vi "test json to variant bool.vi"(8 "error in (no error)":errorcluster) -> (0 "error out":errorcluster)   [LabVIEW 2019, in "labview_json_tests.lvlib"]
uses:
  labview_json_tests.lvlib
  lib/labview_json.lvlib
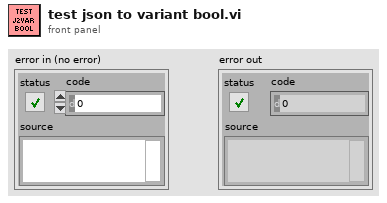
[diagram p1: front panel]
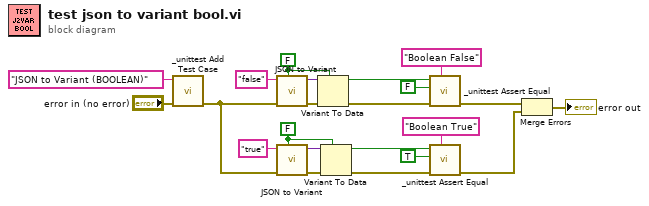
[diagram p0: block diagram]
diagram:
  w2 = FALSE
  w5 = FALSE
  n1 = call "_unittest Add Test Case.vi"("error in (no error)"="error in (no error)", "Test Case"="JSON to Variant (BOOLEAN)") -> ("error out"=w10:errorcluster)  [unwired: 9 in]
  n2 = call "JSON to Variant.vi"("Variant Type"=w5, "error in (no error)"=w10, "JSON"="false") -> ("error out"=w8:errorcluster, "Variant out"=w16:variant)  [unwired: 7 in]
  n3 = call "JSON to Variant.vi"("Variant Type"=w2, "error in (no error)"=w10, "JSON"="true") -> ("error out"=w12:errorcluster, "Variant out"=w3:variant)  [unwired: 7 in]
  n4 = Variant To Data(error in=w8, type=w5, Variant=w16) -> (data=w6:bool, error out=w7:errorcluster)
  n5 = Variant To Data(error in=w12, type=w2, Variant=w3) -> (data=w1:bool, error out=w4:errorcluster)
  n6 = call "_unittest Assert Equal.vi"("Message"="Boolean False", "error in (no error)"=w7, "Expected Value"=FALSE, "Actual Value"=w6) -> ("error out"=w20:errorcluster)  [unwired: 7 in]
  n7 = call "_unittest Assert Equal.vi"("Message"="Boolean True", "error in (no error)"=w4, "Expected Value"=TRUE, "Actual Value"=w1) -> ("error out"=w9:errorcluster)  [unwired: 7 in]
  n8 = Merge Errors(w20, w9) -> (→"error out":errorcluster)
